vi "Destroy User Event.vi"(8 "error in (no error)":errorcluster) -> (0 "error out":errorcluster)   [LabVIEW 2017]
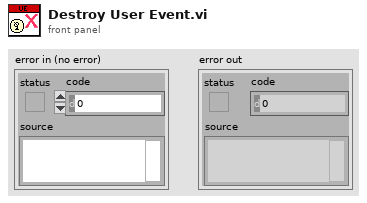
[diagram p1: front panel]
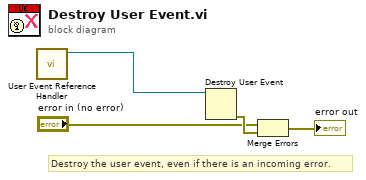
[diagram p0: block diagram]
diagram:
  # "Destroy the user event, even if there is an incoming error."
  n1 = call "User Event Reference Handler.vi"() -> ("User Event Refnum Out"=w1:refnum<user-event>)  [unwired: 9 in, 2 out]
  n2 = Destroy User Event(user event=w1) -> (error out=w4:errorcluster)  [unwired: 1 in]
  n3 = Merge Errors("error in (no error)", w4) -> (→"error out":errorcluster)
